vi "1layer_Neuron.vi"(1 "Offset":dbl, 2 "Weights":fxp<+/-,32,8>[](array[numeric]), 3 "Inputs":fxp<+/-,32,8>[](array[numeric])) -> (0 "Output":fxp<+/-,32,8>)   [LabVIEW 2016]
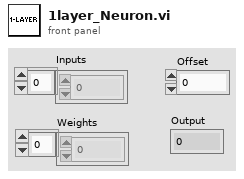
[diagram p1: front panel]
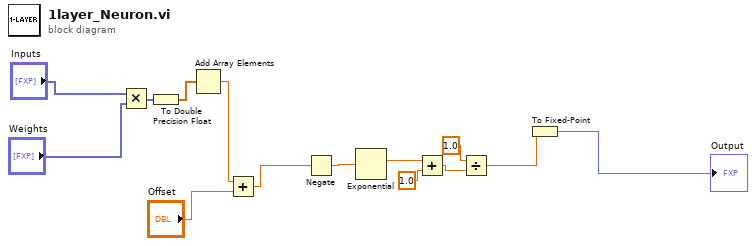
[diagram p0: block diagram]
diagram:
  n1 = Multiply(x="Inputs", y="Weights") -> (x*y=w2:fxp<+/-,64,16>[])
  n2 = To Double Precision Float(number=w2) -> (double precision float=w1:dbl[])
  n3 = Add Array Elements(numeric array=w1) -> (sum=w6:dbl)
  n4 = Add(x=w6, y="Offset") -> (x+y=w5:dbl)
  n5 = Negate(x=w5) -> (-x=w11:dbl)
  n6 = Exponential(1:w11) -> (0:w10:dbl)
  n7 = Add(x=w10, y=1.0) -> (x+y=w13:dbl)
  n8 = Divide(x=1.0, y=w13) -> (x/y=w4:dbl)
  n9 = To Fixed-Point(number=w4) -> (fixed-point=→"Output":fxp<+/-,32,8>)  [unwired: 1 in]
